vi "Reset.vi"(8 "error in":errorcluster, 11 "6700 in":refnum<class "6700.lvclass">) -> (0 "error out":errorcluster, 3 "6700 out":refnum<class "6700.lvclass">)   [LabVIEW 2018, in "6700.lvlib" / "6700.lvclass"]
uses:
  6700.lvclass
  builds/Power_Supply.lvlibp/Power Supply.lvclass
  <instrlib>/Agilent N6700 Series/Agilent N6700 Series.lvlib
  C:/Users/Ron.Dexter.LUMINARTECH/Desktop/builds/Power_Supply.lvlibp/Power Supply.lvclass
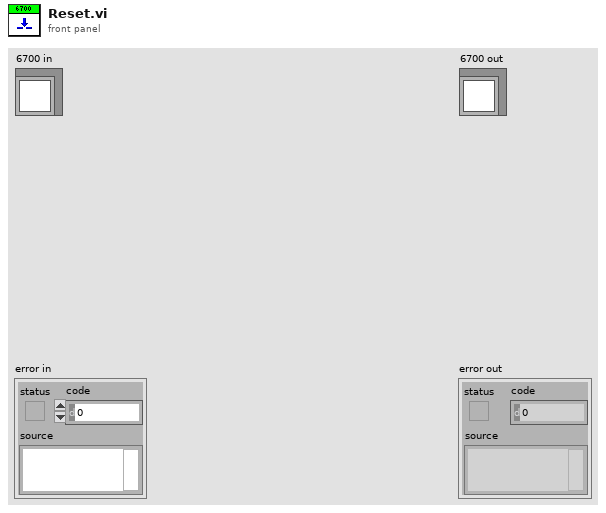
[diagram p1: front panel]
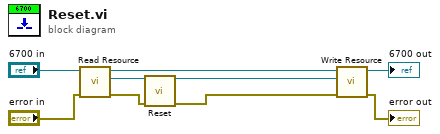
[diagram p0: block diagram]
diagram:
  n1 = call "Read Resource.vi"("error in"="error in", "Power Supply in"="6700 in") -> ("error out"=w7:errorcluster, "Resource"=w8:refnum<visa-resource-name>, "Power Supply out"=w5:refnum<class "6700.lvclass">)  [unwired: 7 in]
  n2 = call <instrlib>:"Reset.vi"("VISA resource name"=w8, "error in (no error)"=w7) -> ("VISA resource name out"=w3:refnum<visa-resource-name>, "error out"=w2:errorcluster)  [unwired: 12 in]
  n3 = call "Write Resource.vi"("error in"=w2, "Resource"=w3, "Power Supply in"=w5) -> ("error out"=→"error out":errorcluster, "Power Supply out"=→"6700 out":refnum<class "6700.lvclass">)  [unwired: 7 in]
